vi "FoodGen.vi"(4 "Time for each food":u16, 5 "Food time in":u16[][](array[numeric]), 6 "Map in":u16[][](array[numeric])) -> (1 "Food time out":u16[][](array[numeric]), 2 "Map out":u16[][](array[numeric]))   [LabVIEW 2014]
doc: "Put a new food into the map. Each food has a count down time.s"
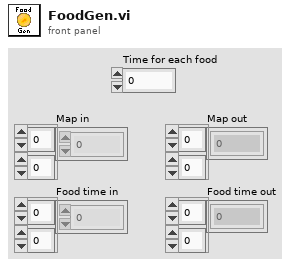
[diagram p1: front panel]
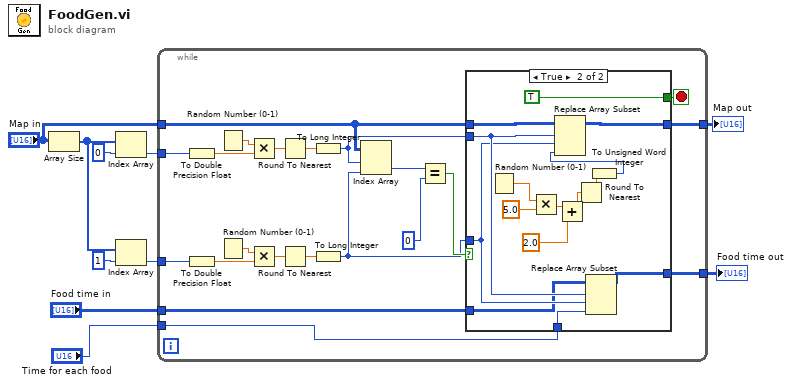
[diagram p0: block diagram]
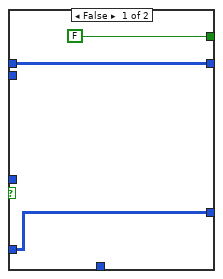
[diagram p2: hidden frame]
diagram:
  n1 = Array Size(array="Map in") -> (size(s)=w7:i32[])
  n2 = Index Array(array=w7, index=0) -> (element=w5:i32)
  n3 = Index Array(array=w7, index=1) -> (element=w4:i32)
  n4 = while {
    tunnel: w5 -> [w30]
    tunnel: w4 -> [w28]
    tunnel: "Map in" -> [w25]
    tunnel: [w21] -> w10
    tunnel: "Food time in" -> [w13]
    tunnel: [w12] -> w1
    tunnel: "Time for each food" -> [w11]
    stop <- w20 stop-if-true
    n5 = To Double Precision Float(number=w30) -> (double precision float=w17:dbl)
    n6 = To Double Precision Float(number=w28) -> (double precision float=w18:dbl)
    n7 = Random Number (0-1)() -> (number: 0 to 1=w16:dbl)
    n8 = Random Number (0-1)() -> (number: 0 to 1=w19:dbl)
    n9 = Multiply(x=w16, y=w17) -> (x*y=w31:dbl)
    n10 = Multiply(x=w19, y=w18) -> (x*y=w29:dbl)
    n11 = Round To Nearest(number=w31) -> (nearest integer value=w24:dbl)
    n12 = Round To Nearest(number=w29) -> (nearest integer value=w23:dbl)
    n13 = To Long Integer(number=w24) -> (32bit integer=w15:i32)
    n14 = To Long Integer(number=w23) -> (32bit integer=w14:i32)
    n15 = Index Array(array=w25, index (row)=w15, index (col)=w14) -> (element=w27:u16)
    n16 = Equal?(x=w27, y=u16 0 ("x")) -> (x = y?=w22:bool)
    n17 = case shown="True" w22 {
      tunnel: w25 -> [w34 w49]
      tunnel: w15 -> [_ w39]
      tunnel: w14 -> [_ w38]
      tunnel: [w34 w48] -> w21
      tunnel: [FALSE TRUE] -> w20
      tunnel: w13 -> [w32 w37]
      tunnel: [w32 w36] -> w12
      tunnel: w11 -> [_ w35]
      frame False {
      }
      frame True {
        n18 = Random Number (0-1)() -> (number: 0 to 1=w46:dbl)
        n19 = Multiply(x=w46, y=5.0) -> (x*y=w44:dbl)
        n20 = Add(x=w44, y=2.0) -> (x+y=w42:dbl)
        n21 = Round To Nearest(number=w42) -> (nearest integer value=w41:dbl)
        n22 = Replace Array Subset(array=w37, new element=w35, index (row)=w39, index (col)=w38) -> (w36:u16[][])
        n23 = To Unsigned Word Integer(number=w41) -> (unsigned 16bit integer=w40:u16)
        n24 = Replace Array Subset(array=w49, new element=w40, index (row)=w39, index (col)=w38) -> (w48:u16[][])
      }
    }
  }
  "Map out" <- w10
  "Food time out" <- w1
